vi "Read States Map.vi"(11 "Debug State Analyzer in":refnum<class "Debug State Analyzer.lvclass">) -> (2 "State Map":map{string, string}(c390), 3 "Debug State Analyzer out":refnum<class "Debug State Analyzer.lvclass">)   [LabVIEW 2020, in "Debug State Analyzer.lvclass"]
uses:
  Debug State Analyzer.lvclass
  Debug State Analyzer.lvclass/Debug State Analyzer.ctl
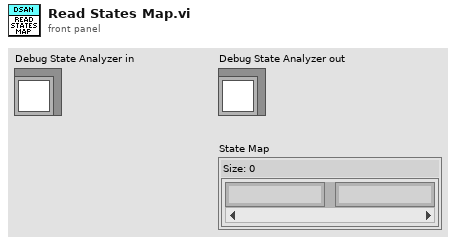
[diagram p1: front panel]
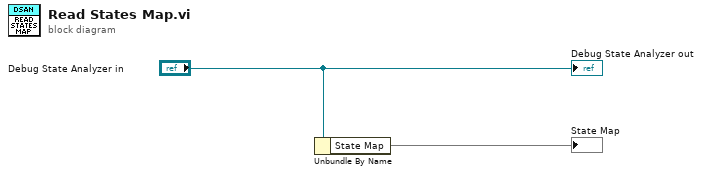
[diagram p0: block diagram]
diagram:
  n1 = Unbundle By Name("Debug State Analyzer in") -> ("State Map"=→"State Map":map{string, string})
  "Debug State Analyzer out" <- "Debug State Analyzer in"
